vi "Parse Data JSON.vi"(8 "error in (no error)":errorcluster, 10 "Data JSON":string, 11 "Server Message in":refnum<class "Server Message.lvclass">) -> (0 "error out":errorcluster, 1 "Replaced?":bool, 2 "Typed Message":refnum<class "Response.lvclass">, 3 "Server Message out":refnum<class "Server Message.lvclass">)   [LabVIEW 2022 SP3, in "obs-websocket-lv.lvlib" / "Server Message.lvclass"]
uses:
  Server Message.lvclass
  Server Message.lvclass/Server Message.ctl
  Response/Response.lvclass
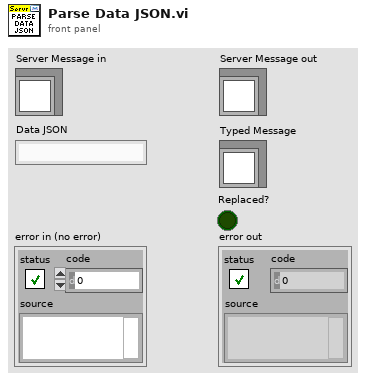
[diagram p1: front panel]
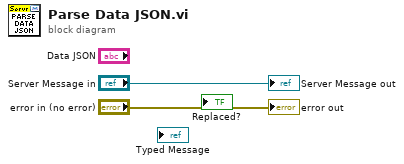
[diagram p0: block diagram]
diagram:
  "error out" <- "error in (no error)"
  "Server Message out" <- "Server Message in"
